vi "tb_4 I16 Array Shifter.vi"() -> ()   [LabVIEW 2011]
panel:
  in  "Trig Offset":u8=1
  out "Output Data":i16[][](array[numeric])
  # "1 2 3 4 in second row"
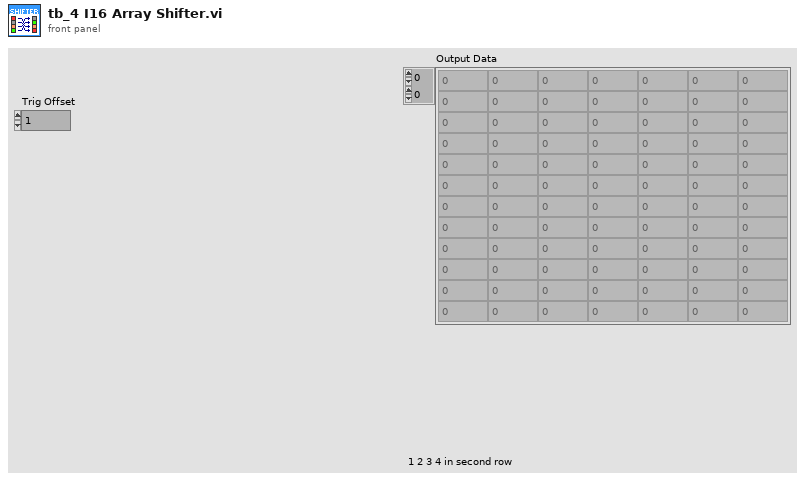
[diagram p1: front panel]
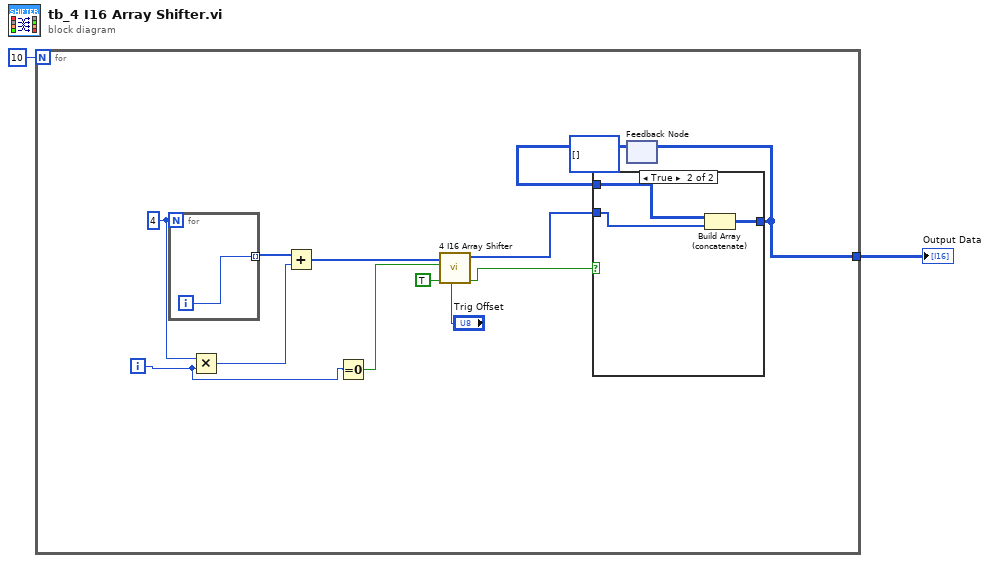
[diagram p0: block diagram]
diagram:
  n1 = for {
    N: 10 -> [_]
    tunnel: [w3] -> w2
    i -> [w8]
    w11 = 4
    n2 = for {
      N: w11 -> [_]
      tunnel: [w20] -> w12 mode=indexing
      i -> [w20]
    }
    n3 = Multiply(x=w11, y=w8) -> (x*y=w10:i32)
    n4 = Add(x=w12, y=w10) -> (x+y=w9:i32[])
    n5 = Equal To 0?(x=w8) -> (x = 0?=w15:bool)
    n6 = call <userlib>:"4 I16 Array Shifter.vi"("Trig Offset"="Trig Offset", "Input Valid"=TRUE, "Start of Read"=w15, "Input Data"=w9) -> ("Output Data Valid"=w7:bool, "Output Data"=w6:i16[])  [unwired: 6 in]
    n7 = feedback #1(i16[][] []) -> (w5:i16[][])
    n8 = case shown="True" w7 {
      tunnel: w6 -> [_ w19]
      tunnel: w5 -> [w16 w18]
      tunnel: [w16 w17] -> w3
      frame False {
      }
      frame True {
        n9 = Build Array (concatenate)(w18, w19) -> (w17:i16[][])
      }
    }
    n10 = feedback-in #1(w3) -> ()
  }
  "Output Data" <- w2
